vi "Bundle_Adjust Text to Fit Rectangle.vi"(0 "VI Name":string, 5 "Number of Rows":i32, 7 "Text settings":T2={"Font"="Small Fonts", "Alignment"=1, "Size"=9, "Center text"=TRUE, "Capitalize text"=TRUE, "Text color"={"Line 1 color"=0, "Line 2 color"=0, "Line 3 color"=0, "Line 4 color"=0}} {"Alignment" items=["left", "center", "right"]}, 9 "Blank Line 1 text?":bool, 11 "Header?":bool) -> (4 "Text out":T1)   [LabVIEW 2025]
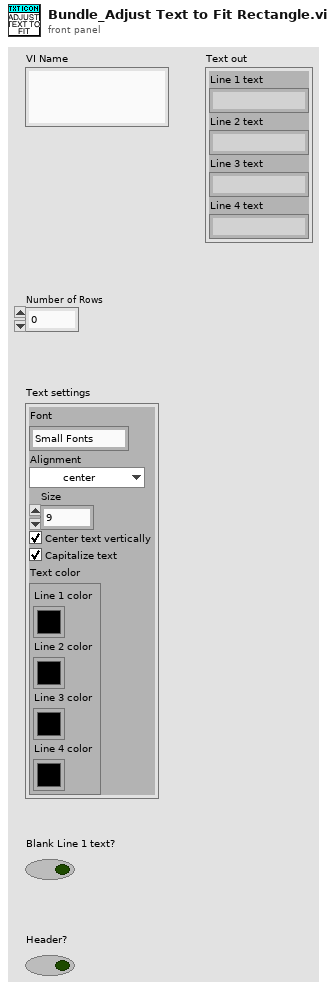
[diagram p1: front panel]
types:
  T1 = cluster{"Line 1 text":string, "Line 2 text":string, "Line 3 text":string, "Line 4 text":string}
  T2 = cluster{"Font":string, "Alignment":u16, "Size":u8, "Center text":bool, "Capitalize text":bool, "Text color":cluster{"Line 1 color":u32, "Line 2 color":u32, "Line 3 color":u32, "Line 4 color":u32}}
  T3 = cluster{"Font Name:":string, "Size":i16, "Strikeout?":bool, "Italic?":bool, "Underline?":bool, "Outline?":bool, "Shadow?":bool, "Bold?":bool}
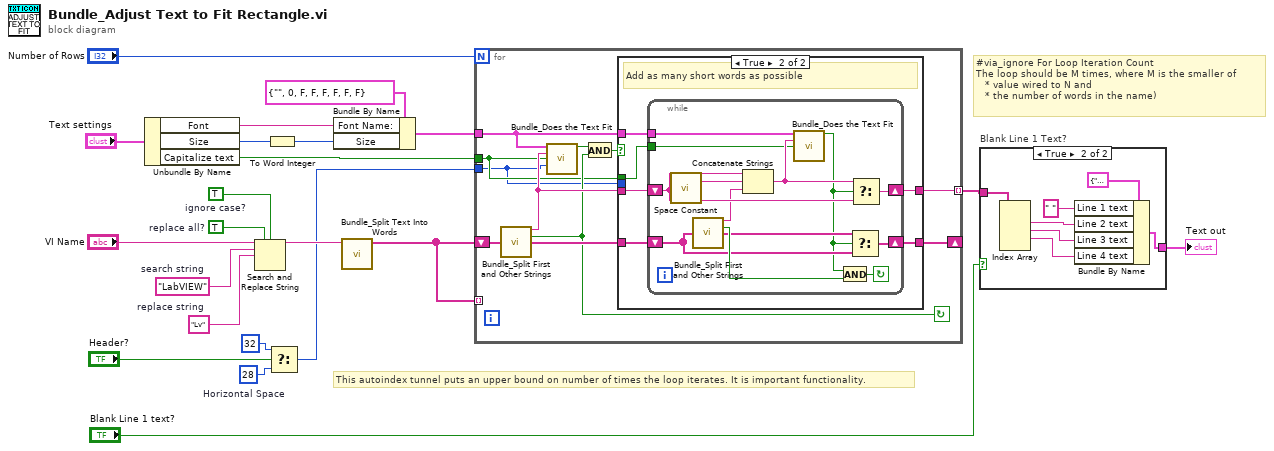
[diagram p0: block diagram]
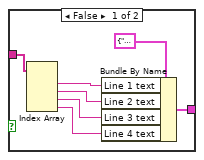
[diagram p2: hidden frame]
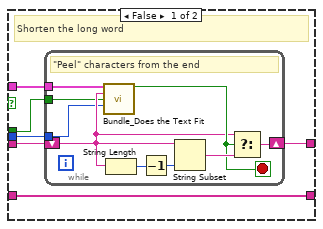
[diagram p3: hidden frame]
diagram:
  w5 = i16 28  # Horizontal Space
  w11 = TRUE  # ignore case?
  w12 = TRUE  # replace all?
  w13 = "Lv"  # replace string
  w14 = "LabVIEW"  # search string
  # "This autoindex tunnel puts an upper bound on number of times the loop iterates. It is important functionality."
  # "#via_ignore For Loop Iteration Count\nThe loop should be M times, where M is the smaller of \n   * value wired to N and \n   * the number of words in the name)"
  n1 = Unbundle By Name("Text settings") -> ("Font"=w20:string, "Size"=w19:u8, "Capitalize text"=w16:bool)
  n2 = Search and Replace String(replace all?=w12, case sensitive?=w11, input string="VI Name", search string=w14, replace string=w13) -> (result string=w9:string)  [unwired: 3 in, 3 out]
  n3 = To Word Integer(number=w19) -> (16bit integer=w17:i16)
  n4 = Select(t=i16 32 ("Horizontal Space"), s="Header?", f=w5) -> (s? t:f=w3:i16)
  n5 = Bundle By Name(cluster=T3 {"Font Name:"="", "Size"=0, "Strikeout?"=FALSE, "Italic?"=FALSE, "Underline?"=FALSE, "Outline?"=FALSE, "Shadow?"=FALSE, "Bold?"=FALSE} ("[user-specified font]"), "Font Name:"=w20, "Size"=w17) -> (w21:T3)
  n6 = call "Bundle_Split Text Into Words.vi"("VI Name"=w9) -> ("Array"=w15:string[])  [unwired: 10 in]
  n7 = for {
    N: "Number of Rows" -> [_]
    tunnel: [w25] -> w7 mode=indexing
    tunnel: w21 -> [w32]
    shift-right: [w33] -> _
    shift-left: w15 -> [w29]
    tunnel: w15 -> [_] mode=indexing
    tunnel: w16 -> [w24]
    tunnel: w3 -> [w23]
    stop <- w26 continue-if-true
    n8 = call "Bundle_Split First and Other Strings.vi"("Strings In"=w29) -> ("First String"=w27:string, "One or More Other Strings"=w26:bool, "Other Strings"=w28:string[])  [unwired: 12 in]
    n9 = call "Bundle_Does the Text Fit.vi"("user-specified font"=w32, "token string"=w27, "Capitalize Text"=w24, "Horizontal Space"=w23) -> ("Text Fits"=w31:bool)  [unwired: 11 in]
    n10 = And(x=w31, y=w26) -> (x .and. y?=w30:bool)
    n11 = case shown="True" w30 {
      tunnel: w32 -> [w36 w54]
      tunnel: w27 -> [w38 w53]
      tunnel: [w37 w52] -> w25
      tunnel: [w39 w51] -> w33
      tunnel: w28 -> [w39 w50]
      tunnel: w24 -> [w35 w49]
      tunnel: w23 -> [w34 _]
      frame False {
        # "Shorten the long word"
        n12 = while {
          shift-right: [w46] -> w37
          shift-left: w38 -> [w42]
          tunnel: w36 -> [w48]
          tunnel: w35 -> [w41]
          tunnel: w34 -> [w40]
          stop <- w45 stop-if-true
          # "\"Peel\" characters from the end"
          n13 = call "Bundle_Does the Text Fit.vi"("user-specified font"=w48, "token string"=w42, "Capitalize Text"=w41, "Horizontal Space"=w40) -> ("Text Fits"=w45:bool)  [unwired: 11 in]
          n14 = String Length(string=w42) -> (length=w44:i32)
          n15 = Decrement(x=w44) -> (x-1=w43:i32)
          n16 = String Subset(string=w42, length (rest)=w43) -> (substring=w47:string)  [unwired: 1 in]
          n17 = Select(t=w42, s=w45, f=w47) -> (s? t:f=w46:string)
        }
      }
      frame True {
        # "Add as many short words as possible"
        n18 = while {
          shift-right: [w67] -> w52
          shift-left: w53 -> [w64]
          tunnel: w54 -> [w66]
          shift-right: [w62] -> w51
          shift-left: w50 -> [w59]
          tunnel: w49 -> [w55]
          stop <- w61 continue-if-true
          n19 = call <vilib>:"Space Constant.vi"() -> ("String"=w65:string)
          n20 = call "Bundle_Split First and Other Strings.vi"("Strings In"=w59) -> ("First String"=w57:string, "One or More Other Strings"=w60:bool, "Other Strings"=w58:string[])  [unwired: 12 in]
          n21 = Concatenate Strings(w64, w65, w57) -> (w63:string)
          n22 = call "Bundle_Does the Text Fit.vi"("user-specified font"=w66, "token string"=w63, "Capitalize Text"=w55) -> ("Text Fits"=w56:bool)  [unwired: 12 in]
          n23 = And(x=w56, y=w60) -> (x .and. y?=w61:bool)
          n24 = Select(t=w58, s=w56, f=w59) -> (s? t:f=w62:string[])
          n25 = Select(t=w63, s=w56, f=w64) -> (s? t:f=w67:string)
        }
      }
    }
  }
  n26 = case "Blank Line 1 Text?" shown="True" "Blank Line 1 text?" {
    tunnel: [w74 w75] -> w1
    tunnel: w7 -> [w69 w77]
    frame False {
      n27 = Index Array(array=w69) -> (element #1=w70:string, element #2=w71:string, element #3=w72:string, element #4=w73:string)  [unwired: 4 in]
      n28 = Bundle By Name(cluster=T1 {"Line 1 text"="", "Line 2 text"="", "Line 3 text"="", "Line 4 text"=""} ("Text out"), "Line 1 text"=w70, "Line 2 text"=w71, "Line 3 text"=w72, "Line 4 text"=w73) -> (w74:T1)
    }
    frame True {
      n29 = Index Array(array=w77) -> (element #1=w79:string, element #2=w80:string, element #3=w81:string)  [unwired: 4 in, 1 out]
      n30 = Bundle By Name(cluster=T1 {"Line 1 text"="", "Line 2 text"="", "Line 3 text"="", "Line 4 text"=""} ("Text out"), "Line 1 text"=" ", "Line 2 text"=w79, "Line 3 text"=w80, "Line 4 text"=w81) -> (w75:T1)
    }
  }
  "Text out" <- w1
